vi "Kalman Filter ().vi"() -> (3 "Observer Library.lvlib:Kalman Filter.lvclass":refnum<class "Kalman Filter.lvclass">)   [LabVIEW 2014, in "Observer Library.lvlib" / "Kalman Filter.lvclass"]
uses:
  Kalman Filter.lvclass
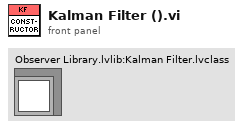
[diagram p1: front panel]
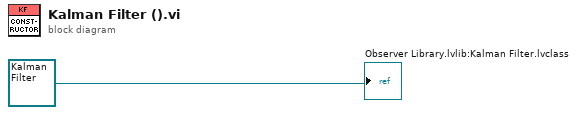
[diagram p0: block diagram]
diagram:
  "Observer Library.lvlib:Kalman Filter.lvclass" <- refnum<class "Kalman Filter.lvclass"> refnum ("Observer Library.lvlib:Kalman Filter.lvclass")
